vi "Probe_Gesture Wrapper.vi"(11 "Message":refnum<class "Channel Message.lvclass">) -> ()   [LabVIEW 2019, in "Gesture Wrapper.lvclass"]
doc: "This VI is used to display information about the message from a channel probe. This VI should never be used as a subVI."
uses:
  Gesture Wrapper.lvclass
  <vilib>/ChannelSupport/Channel Message/Channel Message.lvclass
  e:/builds/penguin/labview/branches/2019/dev/dist/vi.lib/ChannelSupport/Channel Message/Channel Message.lvclass
  Gesture Wrapper.lvclass/Gesture Wrapper.ctl
  <vilib>/ChannelSupport/Channel Message/Channel Message.lvclass/Channel Message.ctl
  Gesture/Gesture.lvclass
panel:
  out "Gesture information":string
  out "Message Class Name":string
  out "Message ID":u32
  # "This probe shows information specific to Gesture Wrapper.lvclass. It was created by following these instructions:\n1. Open this VI:\nvi.lib\\ChannelSupport\\Channel Message\\Probe_Channel Message.vi\n2. Follow the directions on the block diagram of that VI."
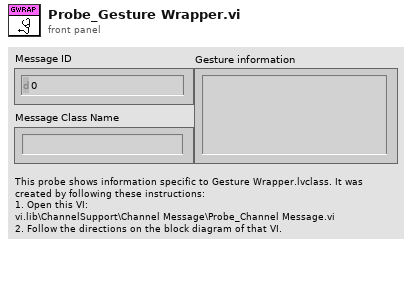
[diagram p1: front panel]
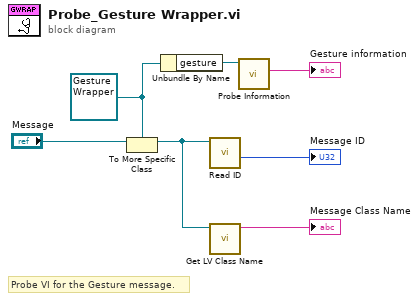
[diagram p0: block diagram]
diagram:
  w3 = refnum<class "Gesture Wrapper.lvclass"> refnum ("Gesture Wrapper")
  # "Probe VI for the Gesture message."
  n1 = To More Specific Class(target class=w3, reference="Message") -> (specific class reference=w4:refnum<class "Gesture Wrapper.lvclass">)  [unwired: 1 in, 1 out]
  n2 = Unbundle By Name(w3) -> ("gesture"=w2:refnum<class "Gesture.lvclass">)
  n3 = call <vilib>:"Read ID.vi"("Channel Message in"=w4) -> ("id"=→"Message ID":u32)  [unwired: 10 in]
  n4 = call <vilib>:"Get LV Class Name.vi"("object"=w4) -> ("class name"=→"Message Class Name":string)  [unwired: 9 in, 1 out]
  n5 = call "Probe Information.vi"("Gesture in"=w2) -> ("probe information"=→"Gesture information":string)  [unwired: 10 in]
